vi "Helper - Populate DataPlugin Settings Listbox.vi"(8 "error in (no error)":errorcluster, 11 "DataPlugins Settings":refnum<vi>) -> (0 "error out":errorcluster)   [LabVIEW 2023]
doc: "Call the List DataPlugins VI to get information on all DataPlugins installed on the system, and populate the DataPlugin Settings listbox with that information."
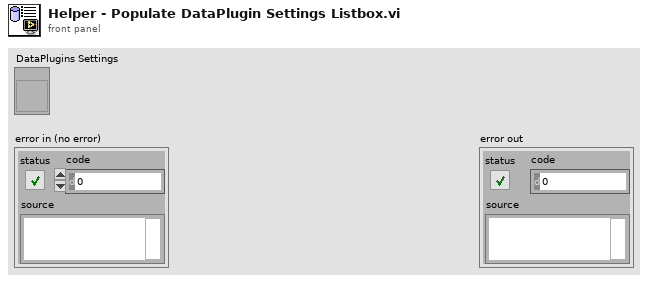
[diagram p1: front panel]
types:
  T1 = typedef "usiPluginInformation.ctl" = cluster{"name":string, "version":string, "type":string, "read-only?":bool, "extensions":string[]}
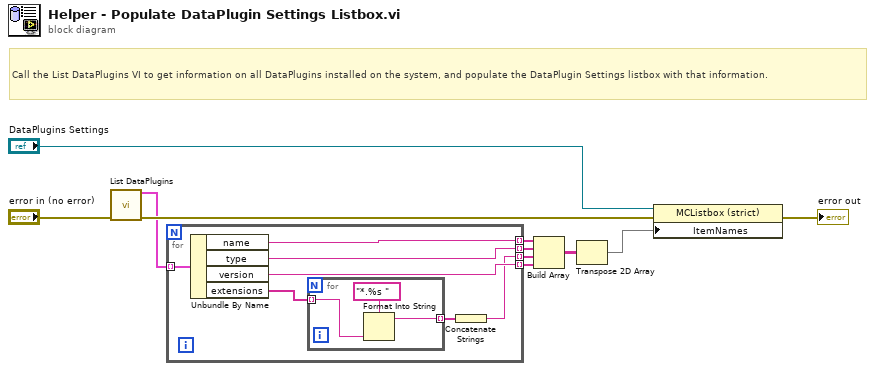
[diagram p0: block diagram]
diagram:
  # "Call the List DataPlugins VI to get information on all DataPlugins installed on the system, and populate the DataPlugin Settings listbox with that information."
  n1 = call <vilib>:"List DataPlugins.vi"("error in (no error)"="error in (no error)") -> ("DataPlugin information"=w4:T1[], "error out"=w5:errorcluster)  [unwired: 13 in]
  n2 = for {
    tunnel: w4 -> [w18] mode=indexing
    tunnel: [w16] -> w3 mode=indexing
    tunnel: [w12] -> w8 mode=indexing
    tunnel: [w15] -> w9 mode=indexing
    tunnel: [w14] -> w10 mode=indexing
    n3 = Unbundle By Name(w18) -> ("name"=w16:string, "type"=w15:string, "version"=w14:string, "extensions"=w17:string[])
    n4 = for {
      tunnel: w17 -> [w20] mode=indexing
      tunnel: [w19] -> w13 mode=indexing
      n5 = Format Into String(format string="*.%s ", w20) -> (resulting string=w19:string)  [unwired: 2 in, 1 out]
    }
    n6 = Concatenate Strings(w13) -> (w12:string)
  }
  n7 = Build Array(w3, w9, w8, w10) -> (w1:string[][])
  n8 = Transpose 2D Array(2D array=w1) -> (transposed array=w2:string[][])
  n9 = property on="Property Node" class="MCListbox (strict)"(reference="DataPlugins Settings", error in=w5, "ItemNames"=w2) -> (error out=→"error out":errorcluster)  [unwired: 1 out]
